vi "RS-232.vi"(5 "Write":bool=TRUE, 6 "read":bool=TRUE, 8 "string to write":string="*IDN?", 10 "bytes to read":u32=5) -> (9 "read string":string)   [LabVIEW 2014]
doc: "The Basic Serial Read and Write example performs a Serial Port Read, a Serial Port Write, or a combination of these actions. The user selects the actions (read or write) on the front panel. If both are selected, the VI will write the data first, read data, and then close the VISA session that is opened to the port. This VI will wait until the specified number of bytes is received at the port. Only the number of bytes specified will be read.\n\nINSTRUCTIONS:\n1) Select the serial resource and configuration parameters (baud rate, data bits, parity, stop bits, flow control).\n2) Select the operations to be performed. \n3) Connect the serial port to your device. If no device is available, perform a loopback test by doing one of the following. Short pins 2 and 3 on a RS-232 cable or short pin 4 to pin 8 and pin 5 to pin 9 on a RS-485/422 cable. \n4) Run the VI to see the data read. (The \"read string\" will match the \"string to write\" if a loopback test was performed.)\n\nNote: The parameters set for the serial port must match the parameters of the connected instrument or device. In this example, the bytes to read parameter specifies the number of bytes that the serial port reads. If there were more bytes at the port than the number specified in bytes to read, those bytes would not be read. Also, if you specify to read more bytes than the number of bytes actually read, you might receive a timeout error message.\n\nOn the block diagram, the Configure Serial Port VI sets the configuration parameters. The front panel displays the controls used to configure the basic parameters, such as baud rate, data bits, and parity. Constants configure the other parameters the user probably does not need set. After the VISA Configure Serial Port VI opens the VISA session and configures the port, the VI passes the VISA resource name to other VIs that perform operations on that VISA resource. The VISA Write function sends a command to the serial device and the VISA Read function returns data based on the command. The VISA Close function then closes the reference to the serial device. It is important to close the reference; otherwise communication through with that port through protocols other than VISA might not be possible."
uses:
  <vilib>/Instr/_visa.llb/VISA Configure Serial Port (Instr).vi
panel:
  in  "Add CheckSum":bool=TRUE
  in  "flow control":u16(ring) items=["None"=0, "XON/XOFF"=1, "RTS/CTS"=2, "DTR/DSR"=4]
  in  "stop bits":u16(ring)=10 items=["1.0"=10, "1.5"=15, "2.0"=20]
  in  "parity":u16(ring) items=["None", "Odd", "Even", "Mark", "Space"]
  in  "data bits":u16=8 min=5 max=8 step=1
  in  "VISA resource name":refnum<visa-resource-name>="COM1"
  in  "baud rate":u32=9600
  in  "Initialize":bool=TRUE
  # "Select the serial resource and the operations (Read, Write, or both) to be performed.  If both are selected, the VI will write the data first, read data and then close the VISA session that is opened to the port.  This VI will wait until the specified number of bytes is received at the port. Only the number of bytes specified will be read."
  # "For additional information select File >> VI Properties >> Documentation"
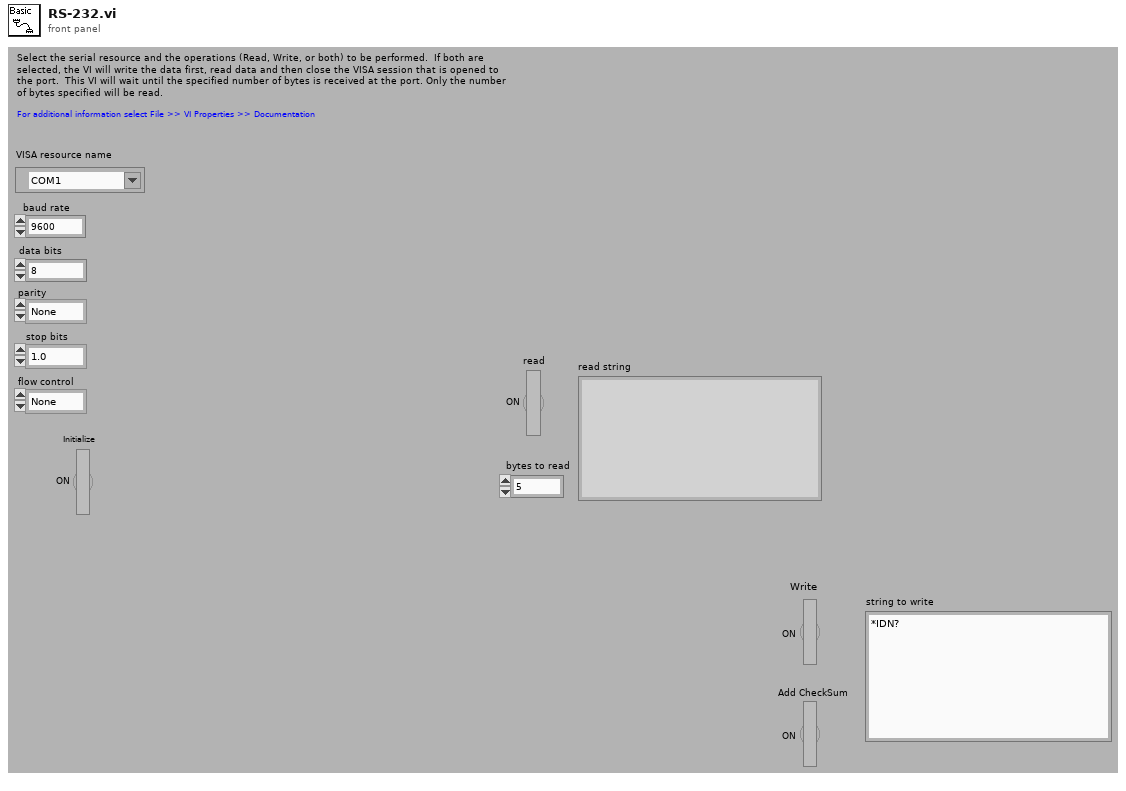
[diagram p1: front panel]
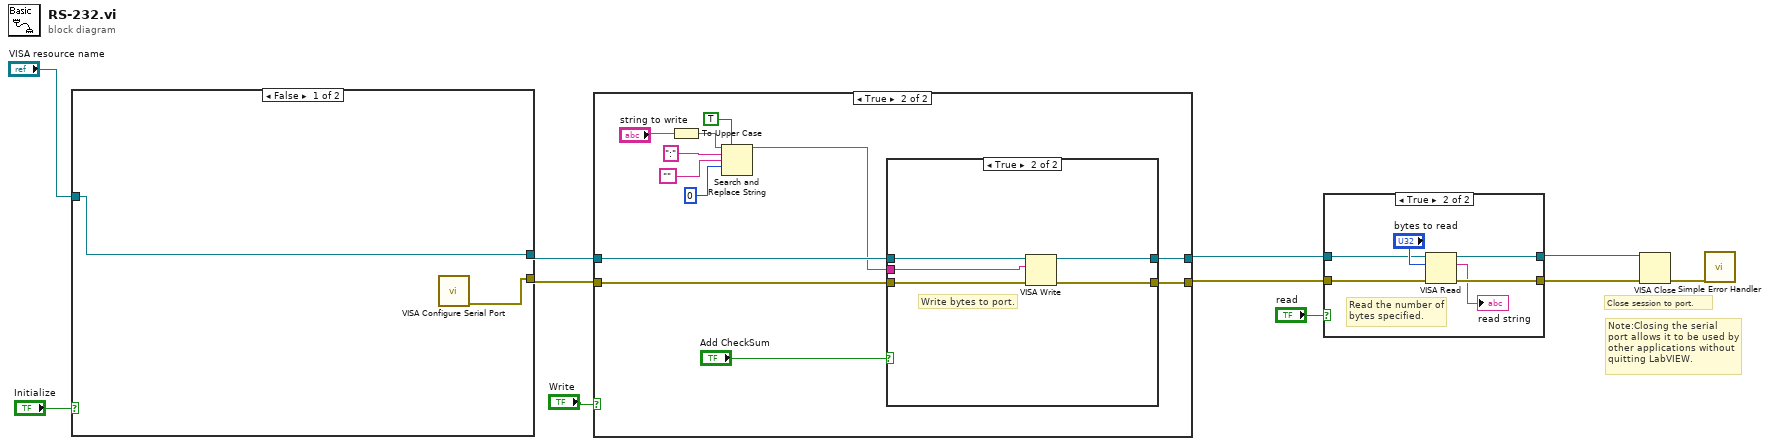
[diagram p0: block diagram]
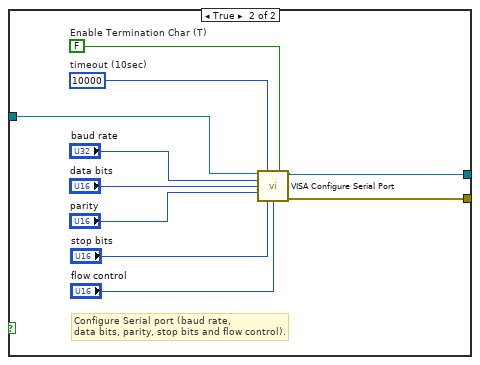
[diagram p2: hidden frame]
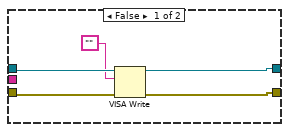
[diagram p4: hidden frame]
diagram:
  # "Note:Closing the serial port allows it to be used by other applications without\nquitting LabVIEW."
  # "Close session to port."
  n1 = case shown="False" "Initialize" {
    tunnel: "VISA resource name" -> [w13 w16]
    tunnel: [w13 w15] -> w2
    tunnel: [w12 w14] -> w1
    frame False {
      n2 = call-poly "VISA Configure Serial Port"() -> ("error out"=w12:errorcluster)  [unwired: 14 in, 1 out]
    }
    frame True {
      w20 = FALSE  # Enable Termination Char (T)
      w21 = u32 10000  # timeout (10sec)
      # "Configure Serial port (baud rate,\ndata bits, parity, stop bits and flow control)."
      n3 = call-poly "VISA Configure Serial Port"("VISA resource name"=w16, "timeout (10sec)"=w21, "Enable Termination\nChar (T)"=w20, "baud rate (9600)"="baud rate", "data bits (8)"="data bits", "parity (0:none)"="parity", "stop bits (10: 1 bit)"="stop bits", "flow control (0:none)"="flow control") -> ("VISA resource name out"=w15:refnum<visa-resource-name>, "error out"=w14:errorcluster)  [unwired: 6 in]
    }
  }
  n4 = case shown="True" "Write" {
    tunnel: [w25 w37] -> w10
    tunnel: w2 -> [w24 w36]
    tunnel: w1 -> [w25 w35]
    tunnel: [w24 w34] -> w5
    frame False {
    }
    frame True {
      n5 = To Upper Case(1:"string to write") -> (0:w31:string)
      n6 = Search and Replace String(replace all?=TRUE ("replace all? (F)"), input string=w31, search string=":", replace string="", offset=0 ("offset (0)")) -> (result string=w26:string)  [unwired: 3 in, 3 out]
      n7 = case shown="True" "Add CheckSum" {
        tunnel: [w41 w47] -> w37
        tunnel: w36 -> [w40 w46]
        tunnel: w35 -> [w39 w45]
        tunnel: [w42 w44] -> w34
        tunnel: w26 -> [_ w43]
        frame False {
          n8 = VISA Write(VISA resource name=w40, write buffer="", error in (no error)=w39) -> (VISA resource name out=w42:refnum<visa-resource-name>, error out=w41:errorcluster)  [unwired: 1 out]
        }
        frame True {
          # "Write bytes to port."
          n9 = VISA Write(VISA resource name=w46, write buffer=w43, error in (no error)=w45) -> (VISA resource name out=w44:refnum<visa-resource-name>, error out=w47:errorcluster)  [unwired: 1 out]
        }
      }
    }
  }
  n10 = case shown="True" "read" {
    tunnel: w10 -> [w49 w52]
    tunnel: [w49 w55] -> w9
    tunnel: [w48 w54] -> w8
    tunnel: w5 -> [w48 w50]
    frame False {
    }
    frame True {
      # "Read the number of bytes specified."
      n11 = VISA Read(VISA resource name=w50, byte count="bytes to read", error in (no error)=w52) -> (VISA resource name out=w54:refnum<visa-resource-name>, read buffer=→"read string":string, error out=w55:errorcluster)  [unwired: 1 out]
    }
  }
  n12 = VISA Close(VISA resource name=w8, error in (no error)=w9) -> (error out=w7:errorcluster)
  n13 = call <vilib>:"Simple Error Handler.vi"("error in (no error)"=w7) -> ()  [unwired: 4 in, 5 out]
